vi "main.vi"() -> ()   [LabVIEW 2019]
uses:
  <vilib>/DAQmx/write.llb/DAQmx Write (Digital Wfm 1Chan NSamp).vi
  <vilib>/DAQmx/write.llb/DAQmx Write (Analog DBL 1Chan 1Samp).vi
  <vilib>/DAQmx/write.llb/DAQmx Write (Digital Bool 1Line 1Point).vi
  <userlib>/AndorSDK3/Data/GetPixelData16.vi
  <vilib>/DAQmx/create/channels.llb/DAQmx Create Channel (AO-Voltage-Basic).vi
  <vilib>/DAQmx/miscellaneous.llb/DAQmx Fill In Error Info.vi
  <vilib>/DAQmx/create/channels.llb/DAQmx Create Channel (DO-Digital Output).vi
  <vilib>/Utility/file.llb/Write Delimited Spreadsheet (DBL).vi
  <vilib>/DAQmx/configure/timing.llb/DAQmx Timing (Sample Clock).vi
  <vilib>/DAQmx/configure/trigger.llb/DAQmx Start Trigger (Digital Edge).vi
  <vilib>/Waveform/DWDTOps.llb/DWDT Uncompress Digital.vi
  <resource>/objmgr/daqmx.rc
panel:
  in  "show temperature":bool
  in  "Start.Retriggerable 2":bool
  in  "waveform generation 3":bool
  out "DO signal 2":dbl[][](array[numeric])
  in  "waveform generation 2":bool
  in  "waveform is generating":bool
  in  "Status":string
  out "acquired images 2":i32
  in  "free run save path":path
  in  "Tab Control 3":enum32{"sCMOS camera"}(tab)
  in  "ExposureTime (s)":dbl=0.1
  in  "PreAmp Gain Control":string(combo)
  in  "Live":bool
  in  "AOI Height":i64
  in  "AOI Width":i64
  in  "Centre AOI":bool
  in  "Apply Settings":bool
  in  "open/close camera":bool
  in  "Trigger mode":string(combo)
  in  "min_value":dbl
  in  "max_value":dbl
  in  "auto constrast":bool
  in  "ElectronicShutteringMode":string(combo)
  in  "Pixel Readout Rate":string(combo)="280 MHz"
  in  "save to disk":bool
  in  "Save path":path
  in  "Frame number":i32
  out "camera temperature(℃)":dbl
  in  "Tab Control 2":enum32{"Control"}(tab)
  out "rps":dbl format="%0.4f"
  in  "Stop/Start":bool
  in  "rotary voltage":dbl min=0.0 max=1.0 step=0.01 format="%0.4f"
  in  "DO Trigger Type":enum32{"No Trigger", "Digital Start"}(ring)
  in  "z position (mm)":dbl min=0.0 max=20.0 step=0.01
  out "T(ms)":dbl format="%0.4f"
  out "camclockfreq":i64
  out "MetaData":i64
  out "TimeStamp":dbl
  in  "Overlap":bool
  out "FrameRate":dbl
  out "get&save image disk":bool
  out "acquired images":i32
  out "dmd_picture_time":dbl
  in  "save parameter":bool
  out "parameters":dbl[](array[numeric])
  in  "Start.Retriggerable":bool
  out "call matlab for acq":bool
  out "call matlab for cali":bool
  out "dmd projection":bool
  out "memory allocated":bool
  in  "waveform generation":bool
  in  "pattern path":path
  in  "load patterns":bool
  in  "get&save image":bool
  out "DO signal":dbl[][](array[numeric])
  in  "String":string
  out "ALP_INVALID_ID":u32=4294967295
  out "saving":bool
  in  "image num":u64
  out "acquiring":bool
  out "previewing":bool
  out "Waveform Graph":dynamicdata(graph)
  out "camera image":T1(plugin-control)
  out "DMD return2":i32[](array[numeric])
  out "DMD return1":i32[](array[numeric])
  out "DMD DevId":u32
  out "DMD SeqId":u32
  in  "initializing":bool
  out "ready":bool
  in  "Error":errorcluster
  out "AOIStride":i64
  out "Pixel Encoding":string
  out "PixelData":u16[](array[numeric])
  out "ByteData":u8[](array[numeric])
  out "ImageSizeBytes":i64
  out "Handle":i32
  in  "z stage COM":refnum<visa-resource-name>
  out "DO sample num":i32=1000
  in  "DO trigger edge":i32(ring)=10280 items=["rising"=10280, "falling"=10171]
  in  "DO trigger channel":tag
  in  "DO channels":tag
  out "DMD pattern":T1(plugin-control)
  in  "Tab Control":enum32{"Free Run", "Calibration", "Acquisition"}(tab)
  in  "free run save":bool caption="Start 2"
  in  "DMD":bool
  in  "File Path":path
  in  "pattern type":u16(ring) items=["from file", "all 0", "all 1"]
  in  "LED":bool
  in  "waveform only":bool
  in  "load cali pattern":bool
  in  "cali pattern path":path
  in  "illumination delay deg":dbl
  in  "start cali":bool
  in  "signal time (ms)":dbl
  in  "cam delay deg":dbl
  in  "dmd delay deg":dbl
  in  "dmd pattern num":u64
  in  "illumination last deg":dbl
  in  "acq signal time (ms)":dbl
  in  "acq waveform only":bool
  in  "acq pattern path":path
  in  "start acq":bool
  in  "rotary in":tag
  in  "starting edge":i32(ring)=10280 items=["Rising"=10280, "Falling"=10171]
  out "sample rate":dbl=1000.0 format="%0.2f"
  in  "counter":tag="Dev1/ctr0"
  in  "rotary out":tag
  in  "Stop":bool
  # "intermediate variables"
  # "indicate that images should be directly saved to disk"
  # "indicate that 'start cali' or 'start acq' has been clicked"
  # "indicate that waveform should be started"
  # "if we want to load patterns on dmd"
  # "how many images will be acquired and saved"
  # "where the cali images and acq images are saved"
  # "where the dmd patterns are loaded"
  # "DO signal that will be generated"
  # "Rotary stage"
  # "Speed monitor"
  # "Z stage"
  # "DMD and camera trigger"
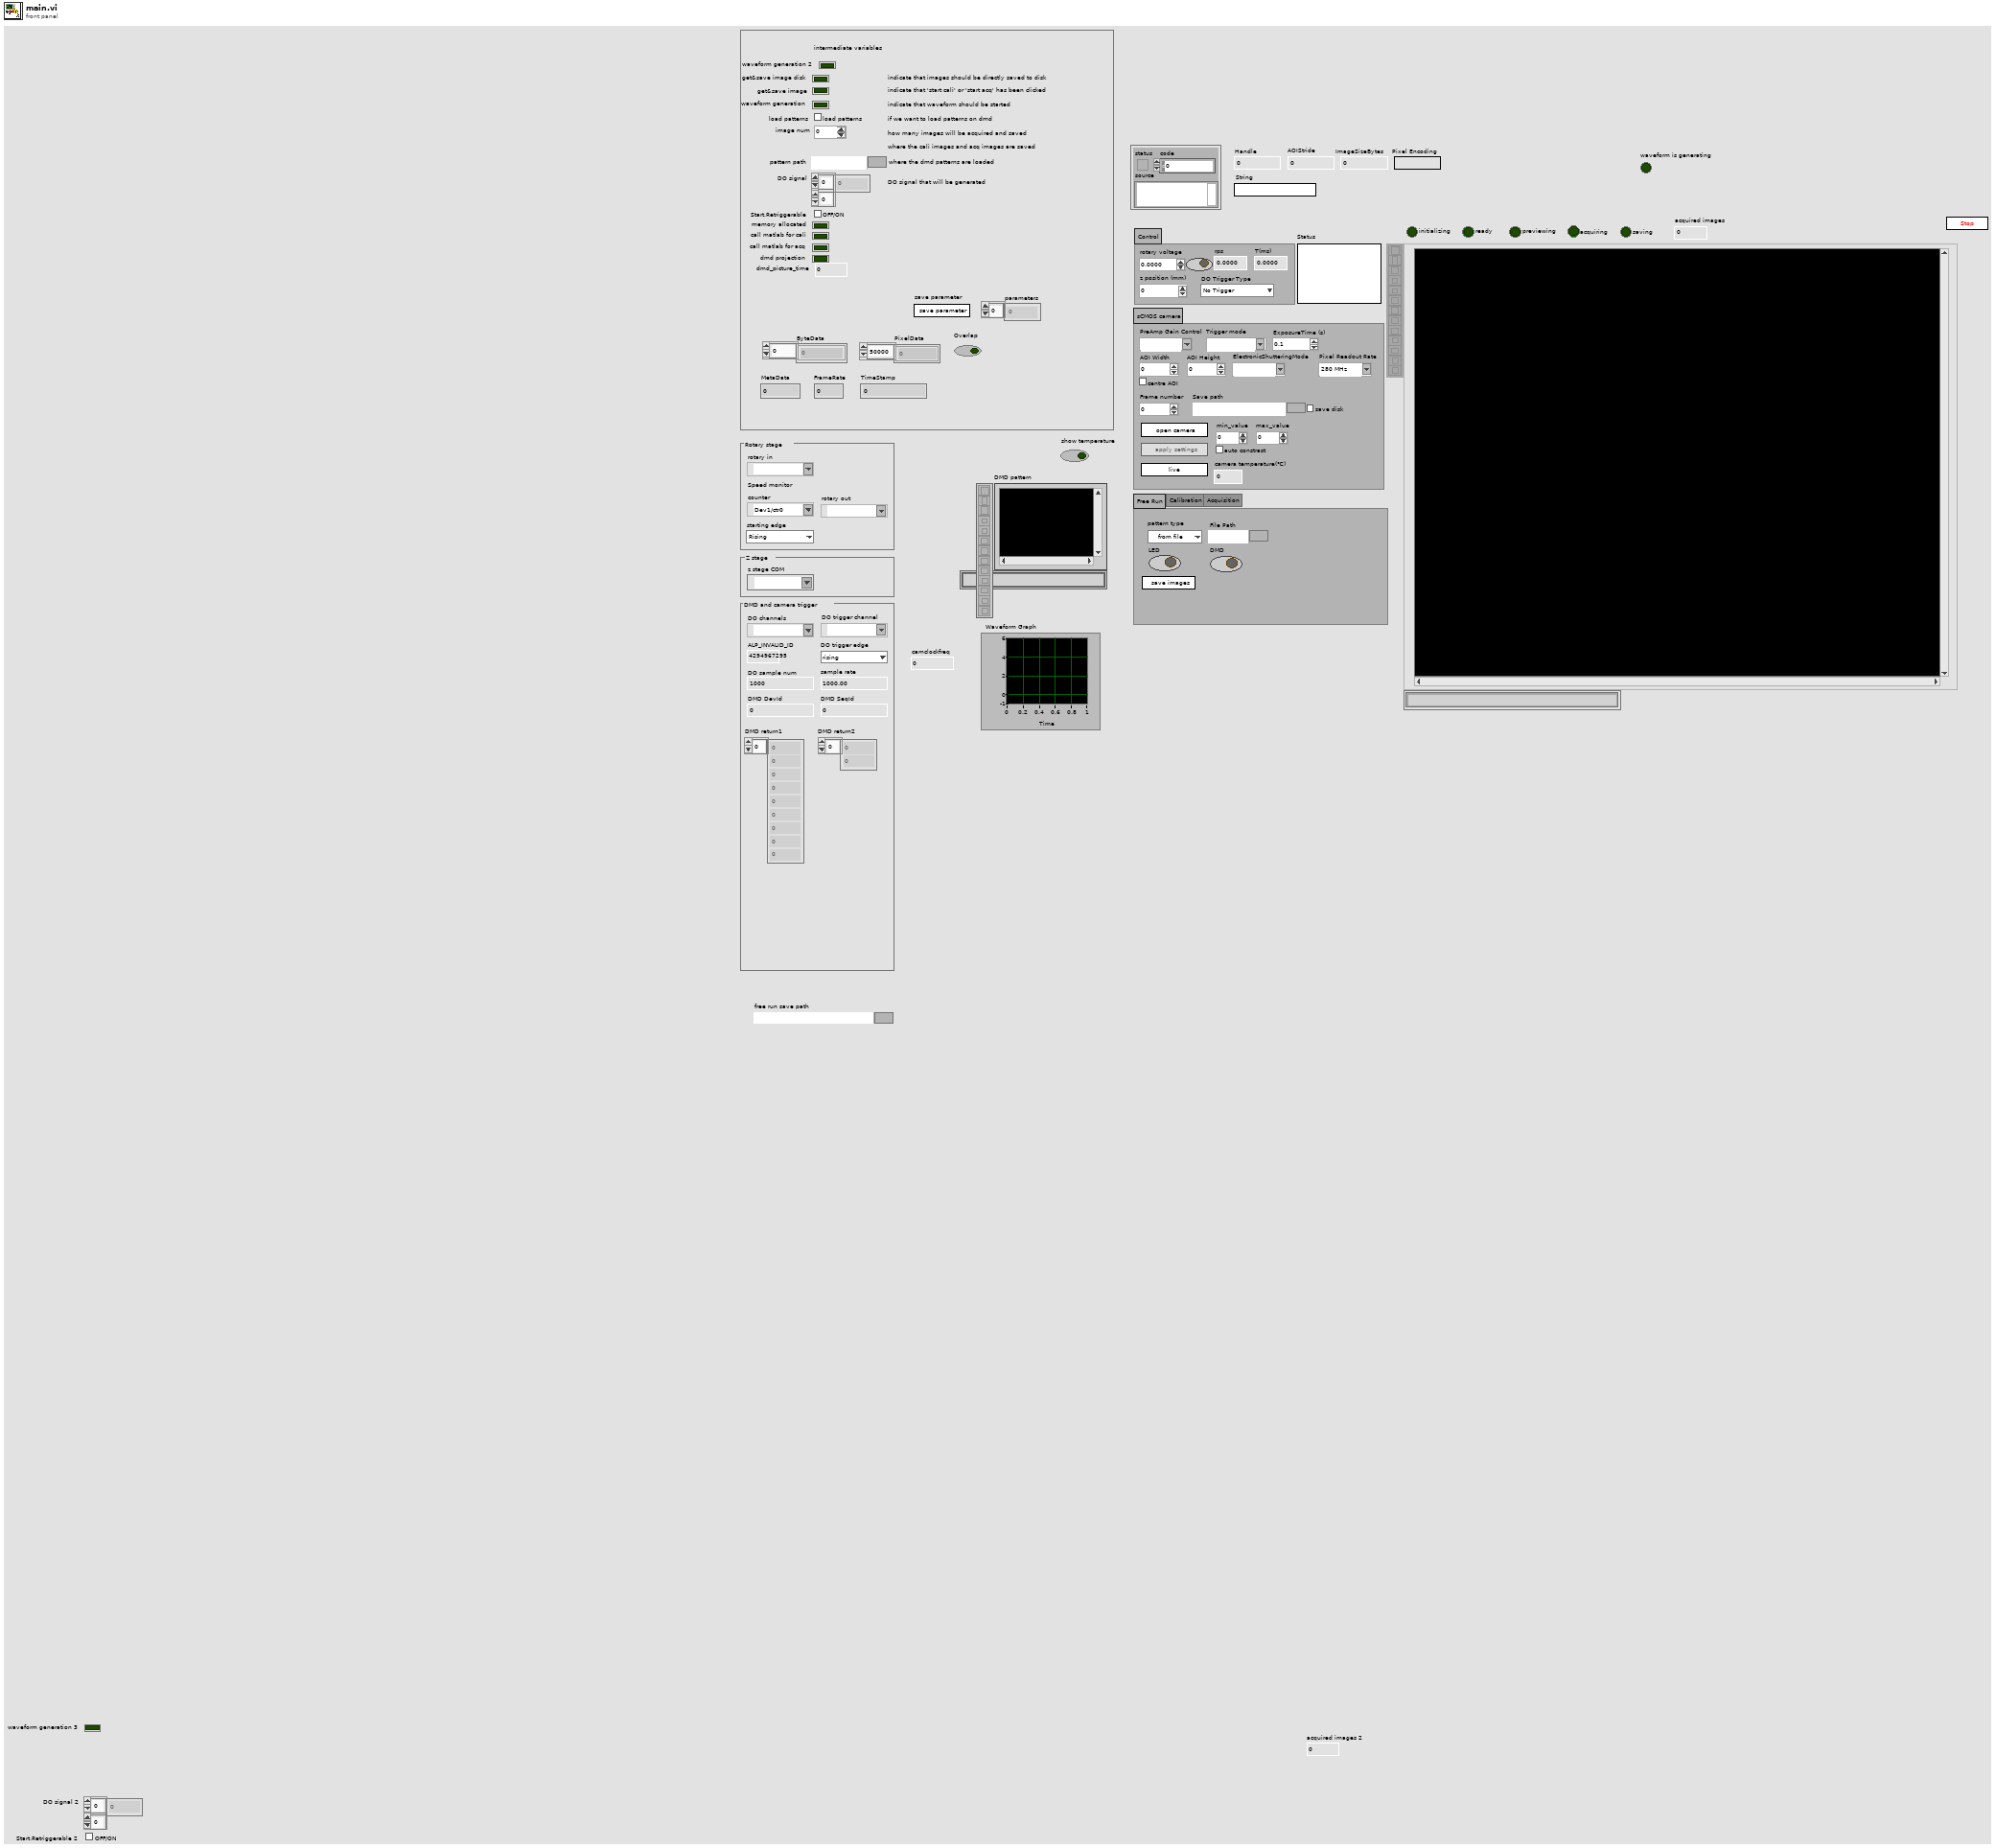
[diagram p1: front panel]
types:
  T1 = typedef "IMAQ Image.ctl" = refnum<image>
  T2 = enum8{"Enabled", "Disabled", "Disabled and Grayed Out"}
  T3 = typedef "Image Type" = u32
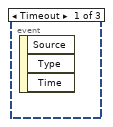
[diagram p3: hidden frame]
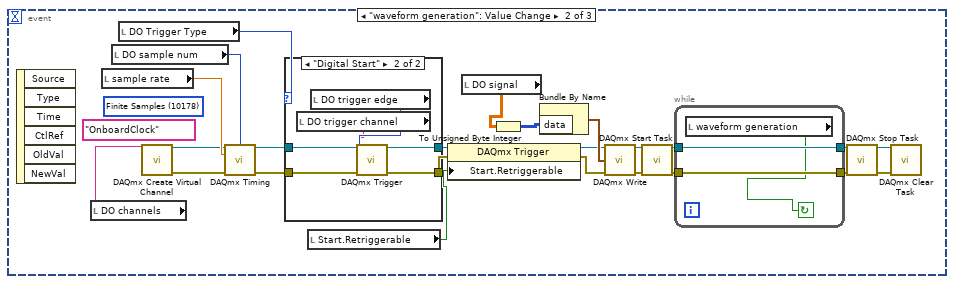
[diagram p4: hidden frame]
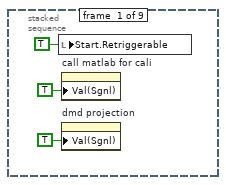
[diagram p7: hidden frame]
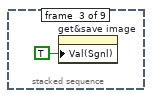
[diagram p8: hidden frame]
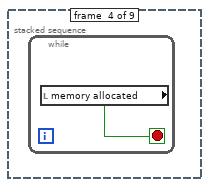
[diagram p9: hidden frame]
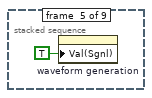
[diagram p10: hidden frame]
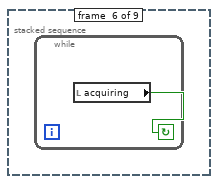
[diagram p11: hidden frame]
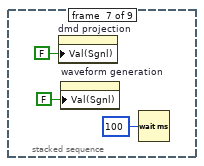
[diagram p12: hidden frame]
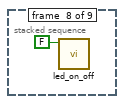
[diagram p13: hidden frame]
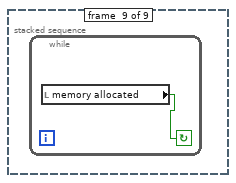
[diagram p14: hidden frame]
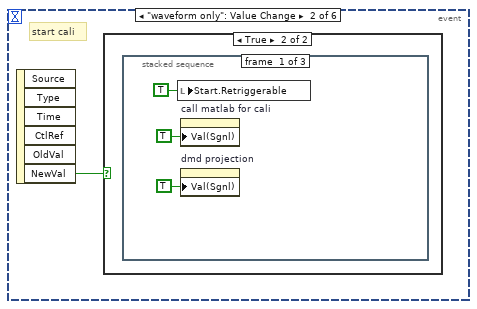
[diagram p15: hidden frame]
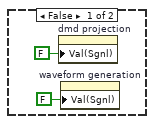
[diagram p16: hidden frame]
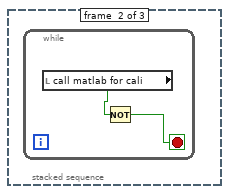
[diagram p17: hidden frame]
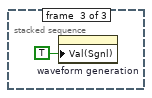
[diagram p18: hidden frame]
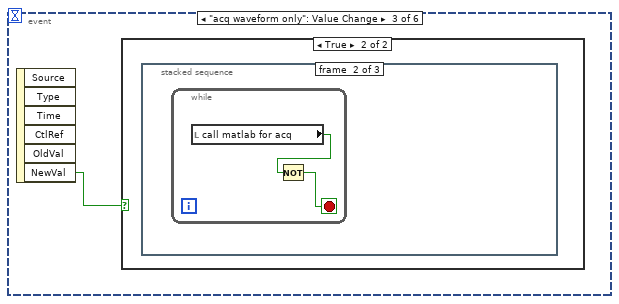
[diagram p19: hidden frame]
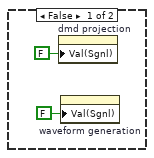
[diagram p20: hidden frame]
diagram:
  n1 = flat-sequence {
    frame #0 {
      w22 = T3 7 items=["Grayscale (U8)", "Grayscale (I16)", "Grayscale (SGL)", "Complex (CSG)", "RGB (U32)", "HSL (U32)", "RGB (U64)", "Grayscale (U16)"] ("Image Type")
      w11 = FALSE ("start button clicked")
      w28 = 10280 items=["rising"=10280, "falling"=10171] ("DO trigger edge")
      w33 = FALSE ("previewing")
      w35 = u16 2 items=["from file", "all 0", "all 1"] ("pattern type")
      w37 = tag "/Dev1/PFI9" ("转台输出通道")
      # "intermediate variables"
      # "acquisition"
      # "gui"
      # "Camera"
      # "Calibration"
      # "free run and dmd"
      # "triggers"
      # "z stage"
      # "rotary stage"
      n2 = Initialize Array(u16 0 ("element"), 2160 ("dimension size"), 2560 ("dimension size")) -> (w17:u16[][])
      n3 = call "IMAQ Create"("Image Name"="cam", "Image Type"=w22) -> ("New Image"=w21:T1)  [unwired: 3 in, 1 out]
      n4 = local read "ALP_INVALID_ID"() -> (w29:u32)
      n5 = call "IMAQ ArrayToImage"("Image Pixels (U16)"=w17, "Image"=w21) -> ("Image Out"=w16:T1)  [unwired: 8 in, 1 out]
      n6 = call <vilib>:"Application Directory.vi"() -> ("Application Directory"=w2:path)
      n7 = call <vilib>:"Application Directory.vi"() -> ("Application Directory"=w3:path)
      n8 = local write "illumination delay deg"(6.0 ("illumination delay deg")) -> ()
      n9 = local write "illumination last deg"(23.0 ("illumination last deg")) -> ()
      n10 = local write "Stop"(FALSE ("停止")) -> ()
      n11 = local write "sample rate"(1000.0 ("采样率")) -> ()
      n12 = local write "Stop/Start"(FALSE ("Stop/Start")) -> ()
      n13 = local write "dmd pattern num"(10.0 ("dmd pattern num")) -> ()
      n14 = local write "pattern type"(w35) -> ()
      n15 = local write "signal time (ms)"(500.0 ("fps")) -> ()
      n16 = Build Path(base path=w3, name or relative path=path "default_image_path/default_save_path" ("cali save path")) -> (appended path=w6:path)
      n17 = Build Path(base path=w2, name or relative path=path "default_image_path/acq_patterns" ("cali pattern path")) -> (appended path=w8:path)
      n18 = local write "z stage COM"(refnum<visa-resource-name> "COM3" ("z stage COM")) -> ()
      n19 = local write "DO trigger edge"(w28) -> ()
      n20 = local write "camera image"(w16) -> ()
      n21 = property on="DMD" class="Bool (strict)"("DisabledEnum"=T2."Enabled" ("Disabled")) -> ()  [unwired: 2 in, 2 out]
      n22 = local write "DO trigger channel"(w37) -> ()
      n23 = local write "cali pattern path"(w8) -> ()
      n24 = local write "rotary out"(w37) -> ()
      n25 = local write "DMD DevId"(w29) -> ()
      n26 = local write "DO Trigger Type"(enum32{"No Trigger", "Digital Start"}."Digital Start" ("DO Trigger Type")) -> ()
      n27 = local write "Save path"(w6) -> ()
      n28 = local write "DO channels"(tag "Dev1/port0/line0:2" ("DO channels")) -> ()
      n29 = local write "rotary in"(tag "Dev1/ao1" ("rotary voltage channel")) -> ()
      n30 = call <vilib>:"Application Directory.vi"() -> ("Application Directory"=w1:path)
      n31 = Build Path(base path=w1, name or relative path=path "default_image_path/acq_patterns" ("cali pattern path")) -> (appended path=w4:path)
      n32 = local write "ExposureTime (s)"(0.01 ("ExposureTime (s)")) -> ()
      n33 = local write "previewing"(w33) -> ()
      n34 = local write "acquiring"(w33) -> ()
      n35 = local write "max_value"(1000.0 ("max_value")) -> ()
      n36 = local write "waveform generation"(w11) -> ()
      n37 = local write "min_value"(0.0 ("min_value")) -> ()
      n38 = local write "Frame number"(10 ("free run frame number")) -> ()
      n39 = local write "get&save image disk"(w11) -> ()
      n40 = local write "show temperature"(FALSE ("show temperature")) -> ()
      n41 = local write "get&save image"(w11) -> ()
      n42 = local write "Tab Control"(enum32{"Free Run", "Calibration", "Acquisition"}."Free Run" ("Tab Control")) -> ()
      n43 = local write "acq pattern path"(w4) -> ()
      n44 = local write "ElectronicShutteringMode"("Global" ("ElectronicShutteringMode")) -> ()
      n45 = local write "Trigger mode"("Software" ("Trigger mode")) -> ()
      "ALP_INVALID_ID" <- u32 4294967295
    }
    frame #1 {
      n46 = while {
        stop <- w52 stop-if-true
        # "waveform for different acquisition"
        n47 = event shown="[2] \"waveform generation 2\": Value Change" {
          selector: _ -> [_ _ _]
          dyn-events: _ -> [_ _ _]
          timeout: 1 -> [_ _ _]
          event Timeout {
            n48 = event-data() -> ()  [unwired: 1 in, 3 out]
          }
          event "waveform generation": Value Change {
            (unwired) 10178 items=["Finite Samples"=10178, "Continuous Samples"=10123, "Hardware Timed Single Point"=12522] ("sample mode")
            (unwired) tag "OnboardClock" ("采样时钟源")
            n49 = event-data() -> ()  [unwired: 1 in, 6 out]
            n50 = local read "DO channels"() -> (w72:tag)
            n51 = local read "sample rate"() -> (w76:dbl)
            n52 = local read "DO sample num"() -> (w75:i32)
            n53 = local read "DO Trigger Type"() -> (w63:enum32{"No Trigger", "Digital Start"})
            n54 = call-poly <vilib>:"DAQmx Create Virtual Channel.vi"("lines"=w72) -> ("task out"=w64:refnum<k21>, "error out"=w65:errorcluster)  [unwired: 13 in]
            n55 = call-poly <vilib>:"DAQmx Timing.vi"("task/channels in"=w64, "samples per channel"=w75, "rate"=w76, "error in"=w65) -> ("task out"=w66:refnum<k21>, "error out"=w67:errorcluster)  [unwired: 10 in]
            n56 = case shown="\"Digital Start\"" w63 {
              tunnel: w66 -> [w81 w87]
              tunnel: w67 -> [w80 w86]
              tunnel: [w81 w85] -> w62
              tunnel: [w80 w84] -> w61
              frame "No Trigger", Default {
              }
              frame "Digital Start" {
                n57 = local read "DO trigger channel"() -> (w82:tag)
                n58 = local read "DO trigger edge"() -> (w83:i32)
                n59 = call-poly <vilib>:"DAQmx Trigger.vi"("task/channels in"=w87, "source"=w82, "edge"=w83, "error in"=w86) -> ("task out"=w85:refnum<k21>, "error out"=w84:errorcluster)  [unwired: 10 in]
              }
            }
            n60 = local read "Start.Retriggerable"() -> (w53:bool)
            n61 = property class="DAQmx Trigger"(reference=w62, error in=w61, "Start.Retriggerable"=w53) -> (reference out=w60:refnum<k21>, error out=w59:errorcluster)
            n62 = local read "DO signal"() -> (w54:dbl[][])
            n63 = To Unsigned Byte Integer(number=w54) -> (unsigned 8bit integer=w73:u8[][])
            n64 = Bundle By Name("data"=w73) -> (w74:digitaldata)  [unwired: 1 in]
            n65 = call-poly <vilib>:"DAQmx Write.vi"("task/channels in"=w60, "data"=w74, "error in"=w59) -> ("task out"=w68:refnum<k21>, "error out"=w69:errorcluster)  [unwired: 10 in, 1 out]
            n66 = call <vilib>:"DAQmx Start Task.vi"("task/channels in"=w68, "error in"=w69) -> ("task out"=w58:refnum<k21>, "error out"=w56:errorcluster)  [unwired: 12 in]
            n67 = while {
              tunnel: w58 -> [w79]
              tunnel: [w79] -> w57
              tunnel: w56 -> [w78]
              tunnel: [w78] -> w55
              stop <- w77 continue-if-true
              n68 = local read "waveform generation"() -> (w77:bool)
            }
            n69 = call <vilib>:"DAQmx Stop Task.vi"("task/channels in"=w57, "error in"=w55) -> ("task out"=w70:refnum<k21>, "error out"=w71:errorcluster)  [unwired: 12 in]
            n70 = call <vilib>:"DAQmx Clear Task.vi"("task in"=w70, "error in"=w71) -> ()  [unwired: 13 in, 1 out]
          }
          event "waveform generation 2": Value Change {
            w98 = 10178 items=["Finite Samples"=10178, "Continuous Samples"=10123, "Hardware Timed Single Point"=12522] ("sample mode")
            n71 = event-data() -> ()  [unwired: 1 in, 6 out]
            n72 = local read "DO channels"() -> (w105:tag)
            n73 = local read "sample rate"() -> (w109:dbl)
            n74 = local read "DO sample num"() -> (w108:i32)
            n75 = call-poly <vilib>:"DAQmx Create Virtual Channel.vi"("lines"=w105) -> ("task out"=w99:refnum<k21>, "error out"=w100:errorcluster)  [unwired: 13 in]
            n76 = call-poly <vilib>:"DAQmx Timing.vi"("task/channels in"=w99, "sample mode"=w98, "samples per channel"=w108, "rate"=w109, "source"=tag "OnboardClock" ("采样时钟源"), "error in"=w100) -> ("task out"=w94:refnum<k21>, "error out"=w93:errorcluster)  [unwired: 8 in]
            n77 = local read "DO signal"() -> (w96:dbl[][])
            n78 = To Unsigned Byte Integer(number=w96) -> (unsigned 8bit integer=w106:u8[][])
            n79 = Bundle By Name("data"=w106) -> (w107:digitaldata)  [unwired: 1 in]
            n80 = call-poly <vilib>:"DAQmx Write.vi"("task/channels in"=w94, "data"=w107, "error in"=w93) -> ("task out"=w101:refnum<k21>, "error out"=w102:errorcluster)  [unwired: 10 in, 1 out]
            n81 = call <vilib>:"DAQmx Start Task.vi"("task/channels in"=w101, "error in"=w102) -> ("task out"=w92:refnum<k21>, "error out"=w91:errorcluster)  [unwired: 12 in]
            n82 = local write "waveform is generating"(TRUE ("Boolean")) -> ()
            n83 = call <vilib>:"DAQmx Wait Until Done.vi"("task/channels in"=w92, "timeout (sec)"=200.0, "error in"=w91) -> ("task out"=w90:refnum<k21>, "error out"=w89:errorcluster)  [unwired: 11 in]
            n84 = call <vilib>:"DAQmx Stop Task.vi"("task/channels in"=w90, "error in"=w89) -> ("task out"=w103:refnum<k21>, "error out"=w104:errorcluster)  [unwired: 12 in]
            n85 = call <vilib>:"DAQmx Clear Task.vi"("task in"=w103, "error in"=w104) -> ()  [unwired: 13 in, 1 out]
          }
        }
        n86 = local read "Stop"() -> (w52:bool)
      }
      n87 = while {
        stop <- w208 stop-if-true
        # "control rotary stage, z stage, free run led, free run dmd, tab change"
        n88 = event shown="[3] \"LED\": Value Change" {
          selector: _ -> [_ _ _ _ _ _ _ _ _]
          dyn-events: _ -> [_ _ _ _ _ _ _ _ _]
          timeout: 1 -> [_ _ _ _ _ _ _ _ _]
          event Timeout {
            n89 = event-data() -> ()  [unwired: 1 in, 3 out]
          }
          event "dmd projection": Value Change {
            n90 = event-data() -> ("NewVal"=w210:bool)  [unwired: 1 in, 5 out]
            n91 = case shown="False" w210 {
              frame False {
                n92 = local read "DMD DevId"() -> (w211:u32)
                n93 = local read "ALP_INVALID_ID"() -> (w213:u32)
                n94 = call "stop_and_free_dmd.vi"("DevId"=w211) -> ("return array2"=w212:i32[])  [unwired: 10 in]
                n95 = local write "DMD return2"(w212) -> ()
                n96 = local write "DMD DevId"(w213) -> ()
              }
              frame True {
                # "project patterns"
                n97 = local read "dmd_picture_time"() -> (w214:dbl)
                n98 = local read "load patterns"() -> (w217:bool)
                n99 = local read "pattern path"() -> (w215:path)
                n100 = call "alloc_and_project_patterns_dmd.vi"("Path"=w215, "PicNum"=10, "load patterns"=w217, "PictureTime"=w214) -> ("return array"=w218:i32[], "SeqId"=w219:u32, "DevId"=w220:u32)  [unwired: 5 in]
                n101 = local write "DMD return1"(w218) -> ()
                n102 = local write "DMD DevId"(w220) -> ()
                n103 = local write "DMD SeqId"(w219) -> ()
              }
            }
          }
          event "rotary voltage": Value Change {
            # "use a AO task to change the stage speed"
            n104 = event-data() -> ()  [unwired: 1 in, 6 out]
            n105 = local read "rotary in"() -> (w222:tag)
            n106 = call <vilib>:"DAQmx Create Task.vi"() -> ("task out"=w233:refnum<k21>, "error out"=w232:errorcluster)  [unwired: 14 in]
            n107 = call-poly <vilib>:"DAQmx Create Virtual Channel.vi"("task in"=w233, "maximum value"=1.0, "minimum value"=0.0, "physical channels"=w222, "error in"=w232) -> ("task out"=w231:refnum<k21>)  [unwired: 9 in, 1 out]
            n108 = local read "rotary voltage"() -> (w221:dbl)
            n109 = call-poly <vilib>:"DAQmx Write.vi"("task/channels in"=w231, "data"=w221) -> ("task out"=w230:refnum<k21>, "error out"=w229:errorcluster)  [unwired: 11 in, 1 out]
            n110 = call <vilib>:"DAQmx Start Task.vi"("task/channels in"=w230, "error in"=w229) -> ("task out"=w228:refnum<k21>, "error out"=w227:errorcluster)  [unwired: 12 in]
            n111 = call <vilib>:"DAQmx Stop Task.vi"("task/channels in"=w228, "error in"=w227) -> ("task out"=w226:refnum<k21>, "error out"=w225:errorcluster)  [unwired: 12 in]
            n112 = call <vilib>:"DAQmx Clear Task.vi"("task in"=w226, "error in"=w225) -> ()  [unwired: 13 in, 1 out]
          }
          event "LED": Value Change {
            w244 = TRUE  # auto start
            # "use DO output to control LED"
            n113 = event-data() -> ()  [unwired: 1 in, 6 out]
            n114 = call <vilib>:"DAQmx Create Task.vi"("auto cleanup"=TRUE) -> ("task out"=w248:refnum<k21>, "error out"=w247:errorcluster)  [unwired: 13 in]
            n115 = call-poly <vilib>:"DAQmx Create Virtual Channel.vi"("task in"=w248, "lines"=tag "Dev1/port0/line2", "error in"=w247) -> ("task out"=w240:refnum<k21>, "error out"=w239:errorcluster)  [unwired: 11 in]
            n116 = call <vilib>:"DAQmx Start Task.vi"("task/channels in"=w240, "error in"=w239) -> ("task out"=w246:refnum<k21>, "error out"=w245:errorcluster)  [unwired: 12 in]
            n117 = local read "LED"() -> (w235:bool)
            n118 = call-poly <vilib>:"DAQmx Write.vi"("task/channels in"=w246, "auto start"=w244, "data"=w235, "timeout"=10.0, "error in"=w245) -> ("task out"=w243:refnum<k21>, "error out"=w242:errorcluster)  [unwired: 8 in, 1 out]
            n119 = call <vilib>:"DAQmx Stop Task.vi"("task/channels in"=w243, "error in"=w242) -> ("task out"=w237:refnum<k21>, "error out"=w238:errorcluster)  [unwired: 12 in]
            n120 = call <vilib>:"DAQmx Clear Task.vi"("task in"=w237, "error in"=w238) -> ()  [unwired: 13 in, 1 out]
          }
          event "DMD": Value Change {
            n121 = event-data() -> ("NewVal"=w249:bool)  [unwired: 1 in, 5 out]
            n122 = case shown="True" w249 {
              frame False {
                n123 = flat-sequence {
                  frame #0 {
                    n124 = local read "DMD DevId"() -> (w251:u32)
                    n125 = call "stop_and_free_dmd.vi"("DevId"=w251) -> ("return array2"=w250:i32[])  [unwired: 10 in]
                    n126 = local write "DMD return2"(w250) -> ()
                  }
                  frame #1 {
                    n127 = local read "ALP_INVALID_ID"() -> (w252:u32)
                    n128 = local write "DMD DevId"(w252) -> ()
                  }
                }
              }
              frame True {
                n129 = local read "pattern type"() -> (w257:u16)
                n130 = local read "File Path"() -> (w258:path)
                n131 = call "alloc_and_project_single_pattern_dmd.vi"("pattern type"=w257, "File Path"=w258) -> ("return array"=w253:i32[], "SeqId"=w254:u32, "DevId"=w255:u32, "Image Out"=w256:T1)  [unwired: 6 in]
                n132 = local write "DMD pattern"(w256) -> ()
                n133 = local write "DMD DevId"(w255) -> ()
                n134 = local write "DMD SeqId"(w254) -> ()
                n135 = local write "DMD return1"(w253) -> ()
              }
            }
          }
          event "save parameter": Value Change {
            n136 = event-data() -> ()  [unwired: 1 in, 6 out]
            n137 = local read "dmd pattern num"() -> (w264:u64)
            n138 = local read "signal time (ms)"() -> (w263:dbl)
            n139 = local read "z position (mm)"() -> (w262:dbl)
            n140 = local read "rotary voltage"() -> (w261:dbl)
            n141 = Build Array(w262, w261, w263, w264) -> (w265:dbl[])
            n142 = call-poly <vilib>:"Write Delimited Spreadsheet.vi"("file path (dialog if empty)"=path "D:/widefield_surface_imaging/parameters.csv", "1D data"=w265, "append to file? (new file:F)"=FALSE) -> ()  [unwired: 11 in, 2 out]
          }
          event "Tab Control": Value Change {
            n143 = event-data() -> ("NewVal"=w269:enum32{"Free Run", "Calibration", "Acquisition"})  [unwired: 1 in, 5 out]
            n144 = local read "ALP_INVALID_ID"() -> (w267:u32)
            n145 = local read "DMD DevId"() -> (w268:u32)
            n146 = case shown="\"Calibration\"" w269 {
              frame "Free Run", Default {
                n147 = local write "Trigger mode"("Software" ("Trigger mode")) -> ()
              }
              frame "Calibration" {
                n148 = local write "save to disk"(FALSE ("save to disk")) -> ()
                n149 = property on="call matlab for cali" class="Bool (strict)"("Val(Sgnl)"=TRUE ("Value (Signaling)")) -> ()  [unwired: 2 in, 2 out]
                n150 = local write "Trigger mode"("External" ("Trigger mode")) -> ()
              }
              frame "Acquisition" {
                n151 = property on="call matlab for acq" class="Bool (strict)"("Val(Sgnl)"=TRUE ("Value (Signaling)")) -> ()  [unwired: 2 in, 2 out]
                n152 = local write "Trigger mode"("External" ("Trigger mode")) -> ()
              }
            }
            n153 = Not Equal?(x=w268, y=w267) -> (x != y?=w266:bool)
            n154 = case shown="True" w266 {
              frame False {
              }
              frame True {
                n155 = local read "DMD DevId"() -> (w272:u32)
                n156 = local read "ALP_INVALID_ID"() -> (w270:u32)
                n157 = call "stop_and_free_dmd.vi"("DevId"=w272) -> ("return array2"=w271:i32[])  [unwired: 10 in]
                n158 = local write "DMD DevId"(w270) -> ()
                n159 = local write "DMD return2"(w271) -> ()
              }
            }
          }
          event "signal time (ms)", "dmd pattern num", "cam delay deg", "dmd delay deg", "illumination last deg", "illumination delay deg": Value Change {
            n160 = event-data() -> ()  [unwired: 1 in, 6 out]
            n161 = property on="call matlab for cali" class="Bool (strict)"("Val(Sgnl)"=TRUE ("Value (Signaling)")) -> ()  [unwired: 2 in, 2 out]
          }
          event "acq signal time (ms)": Value Change {
            n162 = event-data() -> ()  [unwired: 1 in, 6 out]
            n163 = property on="call matlab for acq" class="Bool (strict)"("Val(Sgnl)"=TRUE ("Value (Signaling)")) -> ()  [unwired: 2 in, 2 out]
          }
        }
        n164 = local read "Stop"() -> (w208:bool)
      }
      n165 = while {
        stop <- w281 stop-if-true
        # "preview and get images"
        n166 = event shown="[4] \"get&save image\": Value Change" {
          selector: _ -> [_ _ _ _ _ _]
          dyn-events: _ -> [_ _ _ _ _ _]
          timeout: 1 -> [_ _ _ _ _ _]
          event Timeout {
            n167 = event-data() -> ()  [unwired: 1 in, 3 out]
          }
          event "open/close camera": Value Change {
            n168 = event-data() -> ("NewVal"=w283:bool)  [unwired: 1 in, 5 out]
            n169 = case shown="False" w283 {
              frame False {
                n170 = flat-sequence {
                  frame #0 {
                    n171 = local write "show temperature"(FALSE ("show temperature")) -> ()
                  }
                  frame #1 {
                    # "ShutDown."
                    n172 = local read "Handle"() -> (w285:i32)
                    n173 = call "close_camera.vi"("Handle"=w285) -> ()  [unwired: 11 in]
                  }
                  frame #2 {
                    n174 = local write "ready"(FALSE ("Ready")) -> ()
                    n175 = property on="Apply Settings" class="Bool (strict)"("DisabledEnum"=T2."Disabled and Grayed Out" ("Disabled")) -> ()  [unwired: 2 in, 2 out]
                  }
                }
              }
              frame True {
                n176 = flat-sequence {
                  frame #0 {
                    n177 = call "open_camera.vi"() -> ("error"=w294:errorcluster, "AOI Height"=w293:i64, "AOI Width"=w292:i64, "Handle"=w291:i32, "PreAmp Gain Control"=w295:string)  [unwired: 7 in]
                    n178 = local write "initializing"(TRUE ("Initializing")) -> ()
                    n179 = local write "PreAmp Gain Control"(w295) -> ()
                    n180 = local write "Live"(FALSE ("Run")) -> ()
                    n181 = local write "Handle"(w291) -> ()
                    n182 = local write "AOI Width"(w292) -> ()
                    n183 = local write "AOI Height"(w293) -> ()
                    n184 = local write "Error"(w294) -> ()
                    n185 = property on="Live" class="Bool (strict)"("DisabledEnum"=T2."Disabled and Grayed Out" ("Disabled")) -> ()  [unwired: 2 in, 2 out]
                  }
                  frame #1 {
                    n186 = local write "show temperature"(TRUE ("show temperature")) -> ()
                    n187 = local write "initializing"(FALSE ("Initializing")) -> ()
                    n188 = local write "ready"(TRUE ("Ready")) -> ()
                    n189 = property on="Apply Settings" class="Bool (strict)"("DisabledEnum"=T2."Enabled" ("Disabled")) -> ()  [unwired: 2 in, 2 out]
                  }
                }
              }
            }
          }
          event "Apply Settings": Value Change {
            n190 = event-data() -> ()  [unwired: 1 in, 6 out]
            n191 = flat-sequence {
              frame #0 {
                n192 = local read "ElectronicShutteringMode"() -> (w300:string)
                n193 = local read "PreAmp Gain Control"() -> (w307:string)
                n194 = local read "Trigger mode"() -> (w306:string)
                n195 = local read "ExposureTime (s)"() -> (w312:dbl)
                n196 = local read "Centre AOI"() -> (w308:bool)
                n197 = local read "AOI Height"() -> (w310:i64)
                n198 = local read "AOI Width"() -> (w309:i64)
                n199 = local read "Handle"() -> (w311:i32)
                n200 = call "apply_settings.vi"("Handle"=w311, "PreAmp Gain Control"=w307, "Trigger mode"=w306, "ExposureTime"=w312, "ElectronicShutteringMode"=w300, "AOI Height"=w310, "AOI Width"=w309, "Centre AOI"=w308) -> ("AOIStride"=w305:i64, "ImageSizeBytes"=w304:i64, "Pixel Encoding"=w303:string, "PixelData"=w301:u16[], "ByteData"=w302:u8[])  [unwired: 3 in]
                n201 = local write "AOIStride"(w305) -> ()
                n202 = local write "ImageSizeBytes"(w304) -> ()
                n203 = local write "Pixel Encoding"(w303) -> ()
                n204 = local write "ByteData"(w302) -> ()
                n205 = local write "PixelData"(w301) -> ()
              }
              frame #1 {
                n206 = local write "Apply Settings"(FALSE ("Apply Settings")) -> ()
                n207 = property on="Live" class="Bool (strict)"("DisabledEnum"=T2."Enabled" ("Disabled")) -> ()  [unwired: 2 in, 2 out]
                n208 = local write "ready"(TRUE ("Ready")) -> ()
              }
            }
          }
          event "Live": Value Change {
            n209 = event-data() -> ("NewVal"=w316:bool)  [unwired: 1 in, 5 out]
            n210 = case shown="True" w316 {
              frame False {
                n211 = flat-sequence {
                  frame #0 {
                    # "Stop an acquisition if still running"
                    n212 = local read "Handle"() -> (w318:i32)
                    n213 = call <userlib>:"AT Command A.vi"("Feature"="AcquisitionStop" ("Command"), "Handle"=w318) -> ()  [unwired: 8 in, 2 out]
                  }
                  frame #1 {
                    # "re-enable controls"
                    n214 = local write "previewing"(FALSE ("previewing")) -> ()
                    n215 = property on="Apply Settings" class="Bool (strict)"("DisabledEnum"=T2."Enabled" ("Disabled")) -> ()  [unwired: 2 in, 2 out]
                  }
                }
              }
              frame True {
                w322 = "AcquisitionStart"  # Command
                # "Start the acquisition"
                # "Acquire"
                n216 = local read "Handle"() -> (w324:i32)
                n217 = local read "Error"() -> (w323:errorcluster)
                n218 = call <userlib>:"AT Command A.vi"("error in (no error)"=w323, "Feature"=w322, "Handle"=w324) -> ("error out"=w321:errorcluster)  [unwired: 7 in, 1 out]
                n219 = local write "Error"(w321) -> ()
                n220 = while {
                  tunnel: w324 -> [w328]
                  tunnel: w321 -> [w329]
                  stop <- w327 continue-if-true
                  # "This loop will continiously acquire data from the camera"
                  n221 = flat-sequence {
                    tunnel: w329 -> [w338]
                    tunnel: w328 -> [w339]
                    tunnel: [w330] -> w326
                    tunnel: w326 -> [w344]
                    tunnel: [w343] -> w325
                    tunnel: w325 -> [w353]
                    frame #0 {
                      # "Requeue the buffer\nfor the next image"
                      # "Send a trigger to the camera"
                      # "wait for the acquisition to \nreturn and retrieve the output"
                      n222 = call <userlib>:"AT Command A.vi"("error in (no error)"=w338, "Feature"="SoftwareTrigger" ("Command"), "Handle"=w339) -> ("error out"=w337:errorcluster)  [unwired: 7 in, 1 out]
                      n223 = local write "Error"(w337) -> ()
                      n224 = local read "ImageSizeBytes"() -> (w335:i64)
                      n225 = call <userlib>:"AT Wait Buffer A.vi"("error in (no error)"=w337, "Input buffer"=u32 0, "Timeout"=u32 10000, "Handle"=w339) -> ("error out"=w333:errorcluster, "Output buffer"=w332:u64)  [unwired: 4 in, 2 out]
                      n226 = local write "Error"(w333) -> ()
                      n227 = local read "ByteData"() -> (w336:u8[])
                      n228 = call <userlib>:"PointerToArrayEX.vi"("Array in"=w336, "Pointer In"=w332, "Pointer Size"=w335, "error in (no error)"=w333) -> ("Array out"=w331:u8[], "error out"=w334:errorcluster)  [unwired: 4 in]
                      n229 = local write "ByteData"(w331) -> ()
                      n230 = call <userlib>:"AT Queue Buffer A.vi"("error in (no error)"=w334, "PtrSize"=w335, "Ptr"=w332, "Handle"=w339) -> ("error out"=w330:errorcluster)  [unwired: 6 in, 1 out]
                      n231 = local write "Error"(w330) -> ()
                    }
                    frame #1 {
                      # "Convert the buffer containing byte \ndata into an array of pixels"
                      n232 = local read "Pixel Encoding"() -> (w350:string)
                      n233 = local read "AOI Height"() -> (w347:i64)
                      n234 = local read "AOI Width"() -> (w348:i64)
                      n235 = local read "AOIStride"() -> (w351:i64)
                      n236 = local read "ByteData"() -> (w345:u8[])
                      n237 = local read "PixelData"() -> (w349:u16[])
                      n238 = call-poly <userlib>:"GetPixelData.vi"("Input buffer"=w345, "Output buffer in"=w349, "Pixel Encoding"=w350, "Stride"=w351, "error in (no error)"=w344, "Width"=w348, "Height"=w347) -> ("Output buffer out"=w343:u16[], "error out"=w346:errorcluster)  [unwired: 10 in, 1 out]
                      n239 = local write "Error"(w346) -> ()
                    }
                    frame #2 {
                      w356 = T3 7 items=["Grayscale (U8)", "Grayscale (I16)", "Grayscale (SGL)", "Complex (CSG)", "RGB (U32)", "HSL (U32)", "RGB (U64)", "Grayscale (U16)"] ("Image Type")
                      # "Draw the image"
                      n240 = local read "AOI Height"() -> (w361:i64)
                      n241 = local read "AOI Width"() -> (w360:i64)
                      n242 = local read "auto constrast"() -> (w354:bool)
                      n243 = Reshape Array(w353, w361, w360) -> (w352:u16[][])
                      n244 = case shown="False" w354 {
                        tunnel: [w365 w366] -> w355
                        tunnel: w352 -> [w362 w366]
                        frame False {
                          n245 = local read "min_value"() -> (w364:dbl)
                          n246 = local read "max_value"() -> (w363:dbl)
                          n247 = call "set_min_max.vi"("max_value"=w363, "min_value"=w364, "array_in"=w362) -> ("array_out"=w365:u16[][])  [unwired: 8 in]
                        }
                        frame True {
                        }
                      }
                      n248 = call "IMAQ Create"("Image Name"="cam", "Image Type"=w356) -> ("New Image"=w357:T1)  [unwired: 3 in, 1 out]
                      n249 = call "IMAQ ArrayToImage"("Image Pixels (U16)"=w355, "Image"=w357) -> ("Image Out"=w359:T1)  [unwired: 8 in, 1 out]
                      n250 = local write "camera image"(w359) -> ()
                    }
                  }
                  n251 = local read "Live"() -> (w327:bool)
                  n252 = local write "previewing"(w327) -> ()
                }
              }
            }
          }
          event "get&save image": Value Change {
            n253 = event-data() -> ()  [unwired: 1 in, 6 out]
            n254 = stacked-sequence {
              seq-local: [w370 _ _ _] -> [_ _ w382 _]
              seq-local: [w367 _ _ _] -> [_ _ _ _]
              frame #0 {
                # "allocate memory"
                n255 = local read "image num"() -> (w369:u64)
                n256 = local read "AOI Height"() -> (w373:i64)
                n257 = local read "AOI Width"() -> (w372:i64)
                n258 = Initialize Array(u16 0 ("element"), w369, w373, w372) -> (w370:u16[][][])
                n259 = Initialize Array(0.0 ("element"), w369) -> (w367:dbl[])
              }
              frame #1 {
                n260 = flat-sequence {
                  frame #0 {
                    w379 = "AcquisitionStart"  # Command
                    # "Start the acquisition"
                    n261 = local read "Handle"() -> (w375:i32)
                    n262 = call <userlib>:"AT Command A.vi"("Feature"=w379, "Handle"=w375) -> ("error out"=w378:errorcluster)  [unwired: 8 in, 1 out]
                    n263 = local write "Error"(w378) -> ()
                    n264 = call <userlib>:"AT Get Int A.vi"("error in (no error)"=w378, "Feature"="TimestampClockFrequency", "Handle"=w375) -> ("Value"=w376:i64)  [unwired: 6 in, 2 out]
                    n265 = local write "camclockfreq"(w376) -> ()
                  }
                  frame #1 {
                    n266 = Current VI's Path() -> (path=w380:path)
                    n267 = local write "memory allocated"(TRUE ("memory allocated")) -> ()
                    n268 = call "write_parameteres_to_file1.vi"("vi path"=w380) -> ()  [unwired: 11 in]
                  }
                }
                n269 = local write "acquiring"(TRUE ("acquiring")) -> ()
              }
              frame #2 {
                n270 = local read "Handle"() -> (w383:i32)
                n271 = while {
                  shift-right: [w413] -> w384
                  shift-left: w382 -> [w414]
                  tunnel: w383 -> [w415]
                  i -> [w417]
                  stop <- w412 stop-if-true
                  n272 = stacked-sequence {
                    tunnel: w415 -> [w427 _ _]
                    tunnel: w417 -> [w420 _ w450]
                    tunnel: [_ _ w452] -> w413
                    tunnel: w414 -> [_ _ w451]
                    frame #0 {
                      w423 = u16 24578 items=["MD_FrameData"=24577, "MD_FPGATicks"=24578, "MD_FrameInfo"=24579] ("Metadata Chunk ID")
                      # "Requeue the buffer\nfor the next image"
                      # "wait for the acquisition to \nreturn and retrieve the output"
                      n273 = local read "ImageSizeBytes"() -> (w425:i64)
                      n274 = local read "ByteData"() -> (w430:u8[])
                      n275 = call <userlib>:"AT Wait Buffer A.vi"("Input buffer"=u32 0, "Timeout"=u32 10000, "Handle"=w427) -> ("error out"=w428:errorcluster, "Output buffer"=w426:u64)  [unwired: 5 in, 2 out]
                      n276 = local write "Error"(w428) -> ()
                      n277 = call <userlib>:"PointerToArrayEX.vi"("Array in"=w430, "Pointer In"=w426, "Pointer Size"=w425, "error in (no error)"=w428) -> ("Array out"=w424:u8[], "error out"=w429:errorcluster)  [unwired: 4 in]
                      n278 = local write "ByteData"(w424) -> ()
                      n279 = local read "camclockfreq"() -> (w419:i64)
                      n280 = local read "Save path"() -> (w421:path)
                      n281 = call <userlib>:"AT GetMetadata.vi"("Metadata Chunk ID"=w423, "Input buffer"=w424, "BufferSize"=w425) -> ("MetaData"=w422:i64)  [unwired: 1 in, 2 out]
                      n282 = call "write_timestamp_to_file.vi"("clock freq"=w419, "index"=w420, "metadata"=w422, "free run save path"=w421) -> ()  [unwired: 8 in]
                      n283 = call <userlib>:"AT Queue Buffer A.vi"("error in (no error)"=w429, "PtrSize"=w425, "Ptr"=w426, "Handle"=w427) -> ("error out"=w432:errorcluster)  [unwired: 6 in, 1 out]
                      n284 = local write "Error"(w432) -> ()
                    }
                    frame #1 {
                      # "Convert the buffer containing byte \ndata into an array of pixels"
                      n285 = local read "Pixel Encoding"() -> (w440:string)
                      n286 = local read "AOI Height"() -> (w437:i64)
                      n287 = local read "AOI Width"() -> (w438:i64)
                      n288 = local read "AOIStride"() -> (w441:i64)
                      n289 = local read "ByteData"() -> (w435:u8[])
                      n290 = local read "PixelData"() -> (w439:u16[])
                      n291 = call-poly <userlib>:"GetPixelData.vi"("Input buffer"=w435, "Output buffer in"=w439, "Pixel Encoding"=w440, "Stride"=w441, "Width"=w438, "Height"=w437) -> ("Output buffer out"=w434:u16[], "error out"=w436:errorcluster)  [unwired: 11 in, 1 out]
                      n292 = local write "PixelData"(w434) -> ()
                      n293 = local write "Error"(w436) -> ()
                    }
                    frame #2 {
                      w448 = T3 7 items=["Grayscale (U8)", "Grayscale (I16)", "Grayscale (SGL)", "Complex (CSG)", "RGB (U32)", "HSL (U32)", "RGB (U64)", "Grayscale (U16)"] ("Image Type")
                      # "Draw the image"
                      n294 = local read "ExposureTime (s)"() -> (w443:dbl)
                      n295 = local read "AOI Height"() -> (w454:i64)
                      n296 = local read "AOI Width"() -> (w453:i64)
                      n297 = local read "PixelData"() -> (w455:u16[])
                      n298 = call "IMAQ Create"("Image Name"="1", "Image Type"=w448) -> ("New Image"=w447:T1)  [unwired: 3 in, 1 out]
                      n299 = Reshape Array(w455, w454, w453) -> (w446:u16[][])
                      n300 = call "IMAQ ArrayToImage"("Image Pixels (U16)"=w446, "Image"=w447) -> ("Image Out"=w445:T1)  [unwired: 8 in, 1 out]
                      n301 = Greater?(x=w443, y=0.19) -> (0:w444:bool)
                      n302 = Replace Array Subset(array=w451, new element=w446, index (dim 0)=w450) -> (w452:u16[][][])  [unwired: 2 in]
                      n303 = case shown="True" w444 {
                        tunnel: w445 -> [_ w456]
                        frame False {
                        }
                        frame True {
                          n304 = local write "camera image"(w456) -> ()
                        }
                      }
                    }
                  }
                  n305 = local read "image num"() -> (w411:u64)
                  n306 = Add(x=w417, y=1) -> (x+y=w410:i32)
                  n307 = Greater Or Equal?(x=w410, y=w411) -> (x >= y?=w412:bool)
                  n308 = Not(x=w412) -> (.not. x?=w416:bool)
                  n309 = local write "acquiring"(w416) -> ()
                  n310 = local write "acquired images"(w410) -> ()
                }
                n311 = while {
                  tunnel: w384 -> [w391]
                  i -> [w397]
                  stop <- w392 stop-if-true
                  w394 = T3 7 items=["Grayscale (U8)", "Grayscale (I16)", "Grayscale (SGL)", "Complex (CSG)", "RGB (U32)", "HSL (U32)", "RGB (U64)", "Grayscale (U16)"] ("Image Type")
                  n312 = local read "Save path"() -> (w387:path)
                  n313 = Array Subset(array=w391, index (dim 0)=w397, length (dim 0)=1 ("length")) -> (w407:u16[][][])  [unwired: 4 in]
                  n314 = Add(x=w397, y=1) -> (x+y=w395:i32)
                  n315 = local read "AOI Height"() -> (w406:i64)
                  n316 = local read "AOI Width"() -> (w405:i64)
                  n317 = local read "image num"() -> (w388:u64)
                  n318 = call "IMAQ Create"("Image Name"="2", "Image Type"=w394) -> ("New Image"=w386:T1)  [unwired: 3 in, 1 out]
                  n319 = Path To String(path=w387) -> (string=w390:string)
                  n320 = Format Value(format string="%04d", value (0)=w397) -> (output string=w402:string)  [unwired: 1 in]
                  n321 = Concatenate Strings(w390, "\\" ("string"), w402, ".tif" ("string")) -> (w399:string)
                  n322 = Reshape Array(w407, w406, w405) -> (w404:u16[][])
                  n323 = call "IMAQ ArrayToImage"("Image Pixels (U16)"=w404, "Image"=w386) -> ("error out"=w403:errorcluster, "Image Out"=w385:T1)  [unwired: 8 in]
                  n324 = local write "camera image"(w385) -> ()
                  n325 = Greater Or Equal?(x=w395, y=w388) -> (x >= y?=w392:bool)
                  n326 = Not(x=w392) -> (.not. x?=w393:bool)
                  n327 = String To Path(string=w399) -> (path=w398:path)
                  n328 = local write "saving"(w393) -> ()
                  n329 = call-poly "IMAQ Write File 2"("error in (no error)"=w403, "File Path"=w398, "Image"=w385) -> ()  [unwired: 7 in, 2 out]
                }
              }
              frame #3 {
                w457 = FALSE ("memory allocated")
                # "stop acquisition"
                n330 = local read "Handle"() -> (w459:i32)
                n331 = call <userlib>:"AT Command A.vi"("Feature"="AcquisitionStop" ("Command"), "Handle"=w459) -> ()  [unwired: 8 in, 2 out]
                n332 = local write "memory allocated"(w457) -> ()
                n333 = local write "get&save image"(w457) -> ()
              }
            }
          }
          event "get&save image disk": Value Change {
            n334 = event-data() -> ()  [unwired: 1 in, 6 out]
            n335 = stacked-sequence {
              frame #0 {
                # "Get the AOI Width and Height"
                # "Get Sensor Parameters."
                n336 = local read "Handle"() -> (w463:i32)
                n337 = call <userlib>:"AT Get Int A.vi"("Feature"="AOIHeight" ("Integer feature 2"), "Handle"=w463) -> ("error out"=w462:errorcluster, "Value"=w460:i64)  [unwired: 7 in, 1 out]
                n338 = local write "AOI Height"(w460) -> ()
                n339 = local write "Error"(w462) -> ()
                n340 = call <userlib>:"AT Get Int A.vi"("error in (no error)"=w462, "Feature"="AOIWidth" ("Integer feature"), "Handle"=w463) -> ("error out"=w466:errorcluster, "Value"=w461:i64)  [unwired: 6 in, 1 out]
                n341 = local write "AOI Width"(w461) -> ()
                n342 = local write "Error"(w466) -> ()
              }
              frame #1 {
                # "Set the AOI width and height"
                # "Set the Exposure Time and Pre Amp Gain for the camera"
                # "Set Parameters."
                n343 = local read "ExposureTime (s)"() -> (w480:dbl)
                n344 = local read "Handle"() -> (w467:i32)
                n345 = local read "Error"() -> (w475:errorcluster)
                n346 = call <userlib>:"AT Set Float A.vi"("error in (no error)"=w475, "Value"=w480, "Feature"="ExposureTime" ("ExposureTime"), "Hndl"=w467) -> ("error out"=w478:errorcluster)  [unwired: 6 in, 1 out]
                n347 = local read "PreAmp Gain Control"() -> (w479:string)
                n348 = local write "Error"(w478) -> ()
                n349 = call <userlib>:"AT Set Enum String A.vi"("error in (no error)"=w478, "String"=w479, "Feature"="SimplePreAmpGainControl" ("SimplePreAmpGainControl"), "Handle"=w467) -> ("error out"=w474:errorcluster)  [unwired: 6 in, 1 out]
                n350 = local write "Error"(w474) -> ()
                n351 = local read "AOI Height"() -> (w471:i64)
                n352 = call <userlib>:"AT Set Int A.vi"("error in (no error)"=w474, "Value"=w471, "Feature"="AOIHeight" ("Integer feature"), "Handle"=w467) -> ("error out"=w472:errorcluster)  [unwired: 6 in, 1 out]
                n353 = local write "Error"(w472) -> ()
                n354 = local read "AOI Width"() -> (w470:i64)
                n355 = call <userlib>:"AT Set Int A.vi"("error in (no error)"=w472, "Value"=w470, "Feature"="AOIWidth" ("Integer feature 2"), "Handle"=w467) -> ("error out"=w473:errorcluster)  [unwired: 6 in, 1 out]
                n356 = local write "Error"(w473) -> ()
              }
              frame #2 {
                # "Centre AOI."
                n357 = local read "Centre AOI"() -> (w481:bool)
                n358 = case shown="True" w481 {
                  frame False {
                  }
                  frame True {
                    n359 = local read "AOI Height"() -> (w483:i64)
                    n360 = local read "AOI Width"() -> (w484:i64)
                    n361 = local read "Handle"() -> (w482:i32)
                    n362 = local read "Error"() -> (w485:errorcluster)
                    n363 = call <userlib>:"AT Centre AOI.vi"("error in (no error)"=w485, "AOI Width"=w484, "AOI Height"=w483, "Handle"=w482) -> ("error out"=w486:errorcluster)  [unwired: 7 in]
                    n364 = local write "Error"(w486) -> ()
                  }
                }
              }
              frame #3 {
                # "Set overlap mode,\nfaster frame rates when on"
                # "Set the pixel readout rate"
                # "Set the shutter mode,\nRolling = for fastest frame rate\nGlobal = for fast moving objects"
                # "Set the number of images that \nwill be acquired"
                # "Set the Trigger mode to 'Internal this means \nthis camera will run as fast as possible"
                # "Set the cycle mode to 'Fixed'. This tells the \ncamera to acquire a fixed number of images."
                # "Set Acquisition Mode."
                n365 = local read "Handle"() -> (w493:i32)
                n366 = local read "Error"() -> (w503:errorcluster)
                n367 = call <userlib>:"AT Set Enum String A.vi"("error in (no error)"=w503, "String"="Fixed", "Feature"="CycleMode" ("Enum feature"), "Handle"=w493) -> ("error out"=w502:errorcluster)  [unwired: 6 in, 1 out]
                n368 = local write "Error"(w502) -> ()
                n369 = local read "Trigger mode"() -> (w487:string)
                n370 = call <userlib>:"AT Set Enum String A.vi"("error in (no error)"=w502, "String"=w487, "Feature"="TriggerMode" ("Enum feature"), "Handle"=w493) -> ("error out"=w500:errorcluster)  [unwired: 6 in, 1 out]
                n371 = local write "Error"(w500) -> ()
                n372 = local read "image num"() -> (w498:u64)
                n373 = call <userlib>:"AT Set Int A.vi"("error in (no error)"=w500, "Value"=w498, "Feature"="FrameCount" ("Integer feature 2"), "Handle"=w493) -> ("error out"=w497:errorcluster)  [unwired: 6 in, 1 out]
                n374 = local read "ElectronicShutteringMode"() -> (w490:string)
                n375 = local write "Error"(w497) -> ()
                n376 = call <userlib>:"AT Set Enum String A.vi"("error in (no error)"=w497, "String"=w490, "Feature"="ElectronicShutteringMode" ("ElectronicShutteringMode"), "Handle"=w493) -> ("error out"=w496:errorcluster)  [unwired: 6 in, 1 out]
                n377 = local read "Pixel Readout Rate"() -> (w489:string)
                n378 = call <userlib>:"AT Set Enum String A.vi"("error in (no error)"=w496, "String"=w489, "Feature"="PixelReadoutRate" ("PixelReadoutRate"), "Handle"=w493) -> ("error out"=w495:errorcluster)  [unwired: 6 in, 1 out]
                n379 = local read "Overlap"() -> (w488:bool)
                n380 = call <userlib>:"AT Set Bool A.vi"("error in (no error)"=w495, "Value"=w488, "Feature"="Overlap" ("Overlap"), "Handle"=w493) -> ()  [unwired: 6 in, 2 out]
              }
              frame #4 {
                # "Set Parameters."
                n381 = local read "ExposureTime (s)"() -> (w510:dbl)
                n382 = local read "Handle"() -> (w506:i32)
                n383 = local read "Error"() -> (w507:errorcluster)
                n384 = call <userlib>:"AT Set Float A.vi"("error in (no error)"=w507, "Value"=w510, "Feature"="ExposureTime" ("ExposureTime"), "Hndl"=w506) -> ("error out"=w509:errorcluster)  [unwired: 6 in, 1 out]
                n385 = local write "Error"(w509) -> ()
              }
              frame #5 {
                n386 = local read "Trigger mode"() -> (w511:string)
                n387 = case shown="\"External\", Default" w511 {
                  frame "External", Default {
                    n388 = local read "Handle"() -> (w514:i32)
                    n389 = call <userlib>:"AT Get Float A.vi"("Feature"="FrameRate" ("FrameRate"), "Handle"=w514) -> ("Value"=w512:dbl)  [unwired: 7 in, 2 out]
                    n390 = property on="FrameRate" class="DigNum (strict)"("Value"=w512) -> ()  [unwired: 2 in, 2 out]
                  }
                  frame "Software" {
                    w517 = "FrameRate" ("FrameRate")
                    n391 = local read "Handle"() -> (w516:i32)
                    n392 = call <userlib>:"AT Get Float Max A.vi"("Feature"=w517, "Handle"=w516) -> ("error out"=w520:errorcluster, "MaxValue"=w519:dbl)  [unwired: 7 in, 1 out]
                    n393 = call <userlib>:"AT Set Float A.vi"("error in (no error)"=w520, "Value"=w519, "Feature"=w517, "Hndl"=w516) -> ("error out"=w518:errorcluster)  [unwired: 6 in, 1 out]
                    n394 = call <userlib>:"AT Get Float A.vi"("error in (no error)"=w518, "Feature"=w517, "Handle"=w516) -> ("Value"=w515:dbl)  [unwired: 6 in, 2 out]
                    n395 = property on="FrameRate" class="DigNum (strict)"("Value"=w515) -> ()  [unwired: 2 in, 2 out]
                  }
                  frame "Internal" {
                    w523 = "FrameRate" ("FrameRate")
                    n396 = local read "Handle"() -> (w522:i32)
                    n397 = call <userlib>:"AT Get Float Max A.vi"("Feature"=w523, "Handle"=w522) -> ("error out"=w526:errorcluster, "MaxValue"=w525:dbl)  [unwired: 7 in, 1 out]
                    n398 = call <userlib>:"AT Set Float A.vi"("error in (no error)"=w526, "Value"=w525, "Feature"=w523, "Hndl"=w522) -> ("error out"=w524:errorcluster)  [unwired: 6 in, 1 out]
                    n399 = call <userlib>:"AT Get Float A.vi"("error in (no error)"=w524, "Feature"=w523, "Handle"=w522) -> ("Value"=w521:dbl)  [unwired: 6 in, 2 out]
                    n400 = property on="FrameRate" class="DigNum (strict)"("Value"=w521) -> ()  [unwired: 2 in, 2 out]
                  }
                }
              }
              frame #6 {
                # "Get settings and Create Buffers."
                n401 = stacked-sequence {
                  frame #0 {
                    w535 = "PixelEncoding" ("Enum feature")
                    # "Get the frame rate the camera will run at"
                    # "Retrieve a string containing \nthe current pixel encoding"
                    # "Stride of the\nimage in pixels"
                    # "Size of the\nimages in Bytes.\nHeight*Stride*BytesPerPixel"
                    n402 = local read "Error"() -> (w532:errorcluster)
                    n403 = local read "Handle"() -> (w529:i32)
                    n404 = call <userlib>:"AT Get Int A.vi"("error in (no error)"=w532, "Feature"="AOIStride" ("Integer feature"), "Handle"=w529) -> ("error out"=w538:errorcluster, "Value"=w542:i64)  [unwired: 6 in, 1 out]
                    n405 = call <userlib>:"AT Get Int A.vi"("error in (no error)"=w538, "Feature"="ImageSizeBytes" ("Integer feature"), "Handle"=w529) -> ("error out"=w537:errorcluster, "Value"=w541:i64)  [unwired: 6 in, 1 out]
                    n406 = call <userlib>:"AT Get Enum Index A.vi"("error in (no error)"=w537, "Feature"=w535, "Handle"=w529) -> ("error out"=w536:errorcluster, "Value"=w534:i32)  [unwired: 6 in, 1 out]
                    n407 = call <userlib>:"AT Get Enum String By Index A.vi"("error in (no error)"=w536, "Index"=w534, "Feature"=w535, "Handle"=w529) -> ("error out"=w528:errorcluster, "String"=w533:string)  [unwired: 5 in, 1 out]
                    n408 = call <userlib>:"AT Get Float A.vi"("error in (no error)"=w528, "Feature"="FrameRate", "Handle"=w529) -> ("error out"=w530:errorcluster, "Value"=w527:dbl)  [unwired: 6 in, 1 out]
                    n409 = local write "ImageSizeBytes"(w541) -> ()
                    n410 = local write "Pixel Encoding"(w533) -> ()
                    n411 = local write "AOIStride"(w542) -> ()
                    n412 = local write "Error"(w538) -> ()
                    n413 = local write "Error"(w537) -> ()
                    n414 = local write "Error"(w536) -> ()
                    n415 = local write "Error"(w528) -> ()
                    n416 = local write "FrameRate"(w527) -> ()
                    n417 = local write "Error"(w530) -> ()
                  }
                  frame #1 {
                    w544 = u8 0
                    # "Test for timestamp"
                    # "Buffer to hold the raw data that comes off the camera"
                    n418 = local read "ImageSizeBytes"() -> (w543:i64)
                    n419 = Initialize Array(w544, w543) -> (w545:u8[])
                    n420 = Initialize Array(w544, w543) -> (w546:u8[])
                    n421 = local write "ByteData"(w545) -> ()
                    n422 = local write "PixelData"(w546) -> ()
                  }
                  frame #2 {
                    # "Create 300MB of buffers - this allows sufficient memory to retrieve \ndata into while files are written to disk"
                    # "Clear any buffers \non the camera"
                    n423 = local read "ImageSizeBytes"() -> (w550:i64)
                    n424 = local read "Error"() -> (w557:errorcluster)
                    n425 = local read "Handle"() -> (w555:i32)
                    n426 = Multiply(x=300, y=1024) -> (x*y=w553:i32)
                    n427 = Multiply(x=w553, y=1024) -> (x*y=w549:i32)
                    n428 = call <userlib>:"AT Clear All Buffers A.vi"("error in (no error)"=w557, "Handle"=w555) -> ("error out"=w556:errorcluster)  [unwired: 8 in, 1 out]
                    n429 = local write "Error"(w556) -> ()
                    n430 = Divide(x=w549, y=w550) -> (x/y=w548:dbl)
                    n431 = To Long Integer(number=w548) -> (32bit integer=w547:i32)
                    n432 = for {
                      N: w547 -> [_]
                      tunnel: w556 -> [w560]
                      tunnel: w555 -> [w559]
                      i -> [w558]
                      # "Create a buffer to store 1 image coming off the camera"
                      n433 = local read "ImageSizeBytes"() -> (w562:i64)
                      n434 = call <userlib>:"AT Create Buffer A.vi"("error in (no error)"=w560, "Buffer"=w558, "Size"=w562, "Handle"=w559) -> ("error out"=w563:errorcluster, "Buffer out"=w564:u64)  [unwired: 5 in, 1 out]
                      n435 = local write "Error"(w563) -> ()
                      n436 = call <userlib>:"AT Queue Buffer A.vi"("error in (no error)"=w563, "PtrSize"=w562, "Ptr"=w564, "Handle"=w559) -> ("error out"=w561:errorcluster)  [unwired: 6 in, 1 out]
                      n437 = local write "Error"(w561) -> ()
                    }
                  }
                }
              }
              frame #7 {
                # "2. Queue images as they arrive off the camera"
                # "Acquire"
                n438 = flat-sequence {
                  frame #0 {
                    w570 = "AcquisitionStart"  # Command
                    # "Start the acquisition"
                    n439 = local read "Handle"() -> (w568:i32)
                    n440 = local read "Error"() -> (w571:errorcluster)
                    n441 = call <userlib>:"AT Command A.vi"("error in (no error)"=w571, "Feature"=w570, "Handle"=w568) -> ("error out"=w566:errorcluster)  [unwired: 7 in, 1 out]
                    n442 = Current VI's Path() -> (path=w567:path)
                    n443 = local write "Error"(w566) -> ()
                    n444 = call "write_parameteres_to_file1.vi"("error"=w566, "vi path"=w567) -> ()  [unwired: 10 in]
                    n445 = call <userlib>:"AT Get Int A.vi"("error in (no error)"=w566, "Feature"="TimestampClockFrequency", "Handle"=w568) -> ("Value"=w565:i64)  [unwired: 6 in, 2 out]
                    n446 = local write "camclockfreq"(w565) -> ()
                  }
                  frame #1 {
                    n447 = local write "memory allocated"(TRUE ("memory allocated")) -> ()
                    n448 = local write "acquiring"(TRUE ("acquiring")) -> ()
                  }
                }
              }
              frame #8 {
                n449 = local read "image num"() -> (w574:u64)
                n450 = local read "image num"() -> (w581:u64)
                n451 = local read "Trigger mode"() -> (w580:string)
                n452 = local read "Handle"() -> (w575:i32)
                n453 = Obtain Queue(max queue size (-1, unlimited)=w574, name (unnamed)="Data", element data type=u64 0) -> (queue out=w584:refnum<queue>, error out=w585:errorcluster)  [unwired: 2 in, 1 out]
                n454 = Obtain Queue(max queue size (-1, unlimited)=w581, name (unnamed)="Data", element data type=u64 0) -> (queue out=w583:refnum<queue>)  [unwired: 2 in, 2 out]
                n455 = while {
                  tunnel: w585 -> [w655]
                  tunnel: w584 -> [w654]
                  tunnel: [w651] -> w582
                  i -> [w621]
                  stop <- w644 stop-if-true
                  w637 = T3 7 items=["Grayscale (U8)", "Grayscale (I16)", "Grayscale (SGL)", "Complex (CSG)", "RGB (U32)", "HSL (U32)", "RGB (U64)", "Grayscale (U16)"] ("Image Type")
                  # "3. Write out a file for each image coming off the camera"
                  n456 = local read "ImageSizeBytes"() -> (w645:i64)
                  n457 = Dequeue Element(queue=w654, timeout in ms (-1)=10000, error in (no error)=w655) -> (queue out=w651:refnum<queue>, element=w646:u64, error out=w647:errorcluster)  [unwired: 1 out]
                  n458 = local read "ByteData"() -> (w648:u8[])
                  n459 = local read "Pixel Encoding"() -> (w640:string)
                  n460 = local read "AOI Height"() -> (w633:i64)
                  n461 = local read "AOI Width"() -> (w632:i64)
                  n462 = local read "AOIStride"() -> (w639:i64)
                  n463 = local read "PixelData"() -> (w641:u16[])
                  n464 = call <userlib>:"PointerToArrayEX.vi"("Array in"=w648, "Pointer In"=w646, "Pointer Size"=w645, "error in (no error)"=w647) -> ("Array out"=w642:u8[], "error out"=w620:errorcluster)  [unwired: 4 in]
                  n465 = local read "Save path"() -> (w626:path)
                  n466 = call-poly <userlib>:"GetPixelData.vi"("Input buffer"=w642, "Output buffer in"=w641, "Pixel Encoding"=w640, "Stride"=w639, "error in (no error)"=w620, "Width"=w632, "Height"=w633) -> ("Output buffer out"=w634:u16[], "error out"=w619:errorcluster)  [unwired: 10 in, 1 out]
                  n467 = local read "image num"() -> (w649:u64)
                  n468 = call "IMAQ Create"("Image Name"="s", "Image Type"=w637) -> ("New Image"=w635:T1, "error out"=w636:errorcluster)  [unwired: 3 in]
                  n469 = Reshape Array(w634, w633, w632) -> (w631:u16[][])
                  n470 = Increment(x=w621) -> (x+1=w650:i32)
                  n471 = local read "Handle"() -> (w652:i32)
                  n472 = Path To String(path=w626) -> (string=w630:string)
                  n473 = call "IMAQ ArrayToImage"("Image Pixels (U16)"=w631, "error in (no error)"=w636, "Image"=w635) -> ("Image Out"=w623:T1)  [unwired: 7 in, 1 out]
                  n474 = Format Value(format string="%04d", value (0)=w621) -> (output string=w629:string)  [unwired: 1 in]
                  n475 = Concatenate Strings(w630, "\\" ("string"), w629, ".tif" ("string")) -> (w625:string)
                  n476 = Equal?(x=w650, y=w649) -> (x = y?=w644:bool)
                  n477 = Not(x=w644) -> (.not. x?=w643:bool)
                  n478 = local write "saving"(w643) -> ()
                  n479 = String To Path(string=w625) -> (path=w624:path)
                  n480 = call-poly "IMAQ Write File 2"("File Path"=w624, "Image"=w623) -> ()  [unwired: 8 in, 2 out]
                  n481 = call <userlib>:"AT Queue Buffer A.vi"("error in (no error)"=w619, "PtrSize"=w645, "Ptr"=w646, "Handle"=w652) -> ()  [unwired: 6 in, 2 out]
                }
                n482 = while {
                  tunnel: w575 -> [w599]
                  tunnel: w583 -> [w606]
                  tunnel: w581 -> [w605]
                  tunnel: w580 -> [w601]
                  i -> [w589]
                  stop <- w598 stop-if-true
                  w591 = u16 24578 items=["MD_FrameData"=24577, "MD_FPGATicks"=24578, "MD_FrameInfo"=24579] ("Metadata Chunk ID")
                  n483 = case shown="\"Software\"" w601 {
                    tunnel: [w613 w616 w618] -> w600
                    tunnel: w599 -> [_ w615 _]
                    frame "Internal", Default {
                      n484 = local read "Error"() -> (w613:errorcluster)
                    }
                    frame "Software" {
                      n485 = local read "Error"() -> (w614:errorcluster)
                      n486 = call <userlib>:"AT Command A.vi"("error in (no error)"=w614, "Feature"="SoftwareTrigger" ("Command"), "Handle"=w615) -> ("error out"=w616:errorcluster)  [unwired: 7 in, 1 out]
                    }
                    frame "External" {
                      n487 = local read "Error"() -> (w618:errorcluster)
                    }
                  }
                  n488 = local read "ImageSizeBytes"() -> (w594:i64)
                  n489 = call <userlib>:"AT Wait Buffer A.vi"("error in (no error)"=w600, "Input buffer"=u64 0, "Timeout"=u32 2000, "Handle"=w599) -> ("error out"=w596:errorcluster, "Output buffer"=w602:u64)  [unwired: 4 in, 2 out]
                  n490 = local read "camclockfreq"() -> (w588:i64)
                  n491 = local read "PixelData"() -> (w603:u16[])
                  n492 = local read "Save path"() -> (w587:path)
                  n493 = call <userlib>:"PointerToArrayEX.vi"("Array in"=w603, "Pointer In"=w602, "Pointer Size"=w594, "error in (no error)"=w596) -> ("Array out"=w593:u8[], "error out"=w592:errorcluster)  [unwired: 4 in]
                  n494 = local write "Error"(w596) -> ()
                  n495 = call <userlib>:"AT GetMetadata.vi"("Metadata Chunk ID"=w591, "error in (no error)"=w592, "Input buffer"=w593, "BufferSize"=w594) -> ("MetaData"=w590:i64, "error out"=w586:errorcluster)  [unwired: 1 out]
                  n496 = call "write_timestamp_to_file.vi"("clock freq"=w588, "index"=w589, "metadata"=w590, "free run save path"=w587) -> ()  [unwired: 8 in]
                  n497 = case shown="No Error" w586 {
                    tunnel: w606 -> [w611 _]
                    tunnel: [w610 w612] -> w604
                    tunnel: w602 -> [w609 _]
                    tunnel: w589 -> [w608 _]
                    frame No Error {
                      n498 = Enqueue Element(queue=w611, element=w609) -> ()  [unwired: 2 in, 3 out]
                      n499 = Increment(x=w608) -> (x+1=w610:i32)
                      n500 = local write "acquired images"(w610) -> ()
                    }
                    frame Error {
                      n501 = local read "image num"() -> (w612:u64)
                    }
                  }
                  n502 = Equal?(x=w605, y=w604) -> (x = y?=w598:bool)
                  n503 = Not(x=w598) -> (.not. x?=w597:bool)
                  n504 = local write "acquiring"(w597) -> ()
                }
                n505 = Release Queue(queue=w582) -> ()  [unwired: 2 in, 3 out]
              }
              frame #9 {
                n506 = flat-sequence {
                  frame #0 {
                    # "Stop an acquisition if still running"
                    n507 = local read "Handle"() -> (w657:i32)
                    n508 = call <userlib>:"AT Command A.vi"("Feature"="AcquisitionStop" ("Command"), "Handle"=w657) -> ()  [unwired: 8 in, 2 out]
                  }
                  frame #1 {
                    w658 = FALSE ("get&save image disk")
                    # "Clear any buffers \non the camera"
                    n509 = local read "Error"() -> (w659:errorcluster)
                    n510 = local read "Handle"() -> (w661:i32)
                    n511 = call <userlib>:"AT Clear All Buffers A.vi"("error in (no error)"=w659, "Handle"=w661) -> ("error out"=w660:errorcluster)  [unwired: 8 in, 1 out]
                    n512 = local write "memory allocated"(w658) -> ()
                    n513 = local write "get&save image disk"(w658) -> ()
                    n514 = local write "Error"(w660) -> ()
                  }
                }
              }
            }
          }
        }
        n515 = local read "Stop"() -> (w281:bool)
      }
      n516 = while {
        stop <- w46 stop-if-true
        n517 = local read "show temperature"() -> (w45:bool)
        n518 = case shown="True" w45 {
          frame False {
          }
          frame True {
            n519 = local read "Handle"() -> (w49:i32)
            n520 = call <userlib>:"AT Get Float A.vi"("Feature"="SensorTemperature" ("SensorTemperature"), "Handle"=w49) -> ("Value"=→"camera temperature(℃)":dbl)  [unwired: 7 in, 2 out]
          }
        }
        n521 = local read "Stop"() -> (w46:bool)
        n522 = Wait (ms)(milliseconds to wait=u32 100) -> ()  [unwired: 1 out]
      }
      n523 = while {
        stop <- w175 stop-if-true
        # "matlab related events"
        n524 = event shown="[2] \"call matlab for acq\": Value Change" {
          selector: _ -> [_ _ _]
          dyn-events: _ -> [_ _ _]
          timeout: 1 -> [_ _ _]
          event Timeout {
            n525 = event-data() -> ()  [unwired: 1 in, 3 out]
          }
          event "call matlab for cali": Value Change {
            n526 = event-data() -> ()  [unwired: 1 in, 6 out]
            n527 = stacked-sequence {
              frame #0 {
                n528 = local read "illumination delay deg"() -> (w182:dbl)
                n529 = local read "illumination last deg"() -> (w181:dbl)
                n530 = local read "dmd pattern num"() -> (w183:u64)
                n531 = local read "dmd pattern num"() -> (w177:u64)
                n532 = local read "cali pattern path"() -> (w188:path)
                n533 = local read "load cali pattern"() -> (w187:bool)
                n534 = local read "signal time (ms)"() -> (w184:dbl)
                n535 = local read "Frame number"() -> (w178:i32)
                n536 = local read "dmd delay deg"() -> (w185:dbl)
                n537 = local read "cam delay deg"() -> (w186:dbl)
                n538 = Multiply(x=w178, y=w177) -> (x*y=w176:u64)
                n539 = local write "load patterns"(w187) -> ()
                n540 = local write "pattern path"(w188) -> ()
                n541 = call "matlab_for_calibration.vi"("illumination last degree"=w181, "illumination delay degree"=w182, "dmd pattern num"=w183, "camera delay degree"=w186, "dmd delay degree"=w185, "signal_time(ms)"=w184) -> ("exposure time(s)"=w190:dbl, "sample num"=w191:dbl, "DO signal"=w189:dbl[][], "sample rate"=w180:dbl, "dmd_picture_time(us)"=w179:dbl)  [unwired: 1 in]
                n542 = local write "image num"(w176) -> ()
                n543 = local write "ExposureTime (s)"(w190) -> ()
                n544 = local write "DO signal"(w189) -> ()
                n545 = local write "DO sample num"(w191) -> ()
                n546 = local write "dmd_picture_time"(w179) -> ()
                n547 = local write "sample rate"(w180) -> ()
              }
              frame #1 {
                n548 = local write "call matlab for cali"(FALSE ("call matlab for cali")) -> ()
              }
            }
          }
          event "call matlab for acq": Value Change {
            n549 = event-data() -> ()  [unwired: 1 in, 6 out]
            n550 = stacked-sequence {
              frame #0 {
                n551 = local read "illumination delay deg"() -> (w196:dbl)
                n552 = local read "illumination last deg"() -> (w195:dbl)
                n553 = local read "acq pattern path"() -> (w205:path)
                n554 = local read "acq signal time (ms)"() -> (w198:dbl)
                n555 = local read "dmd pattern num"() -> (w197:u64)
                n556 = local read "Frame number"() -> (w206:i32)
                n557 = local read "dmd delay deg"() -> (w199:dbl)
                n558 = local read "cam delay deg"() -> (w200:dbl)
                n559 = local write "image num"(w206) -> ()
                n560 = local write "load patterns"(TRUE) -> ()
                n561 = local write "pattern path"(w205) -> ()
                n562 = call "matlab_for_acquisition.vi"("illumination last degree"=w195, "illumination delay degree"=w196, "dmd pattern num"=w197, "camera delay degree"=w200, "dmd delay degree"=w199, "signal_time(ms)"=w198) -> ("exposure time"=w201:dbl, "sample num"=w203:dbl, "DO signal"=w202:dbl[][], "sample rate"=w204:dbl, "dmd_picture_time"=w193:dbl)  [unwired: 1 in]
                n563 = local write "DO sample num"(w203) -> ()
                n564 = local write "ExposureTime (s)"(w201) -> ()
                n565 = local write "dmd_picture_time"(w193) -> ()
                n566 = local write "sample rate"(w204) -> ()
                n567 = local write "DO signal"(w202) -> ()
              }
              frame #1 {
                n568 = local write "call matlab for acq"(FALSE ("call matlab for acq")) -> ()
              }
            }
          }
        }
        n569 = local read "Stop"() -> (w175:bool)
      }
      n570 = while {
        stop <- w111 stop-if-true
        n571 = event shown="[0] \"start cali\": Value Change" {
          selector: _ -> [_ _ _ _ _ _]
          dyn-events: _ -> [_ _ _ _ _ _]
          timeout: 1 -> [_ _ _ _ _ _]
          event "start cali": Value Change {
            # "start cali"
            n572 = event-data() -> ()  [unwired: 1 in, 6 out]
            n573 = local read "rotary voltage"() -> (w114:dbl)
            n574 = Greater?(x=w114, y=0.0) -> (0:w112:bool)
            n575 = case shown="True" w112 {
              frame False {
              }
              frame True {
                n576 = stacked-sequence {
                  frame #0 {
                    n577 = local write "Start.Retriggerable"(TRUE ("Start.Retriggerable")) -> ()
                    n578 = property on="call matlab for cali" class="Bool (strict)"("Val(Sgnl)"=TRUE ("Value (Signaling)")) -> ()  [unwired: 2 in, 2 out]
                    n579 = property on="dmd projection" class="Bool (strict)"("Val(Sgnl)"=TRUE ("Value (Signaling)")) -> ()  [unwired: 2 in, 2 out]
                  }
                  frame #1 {
                    n580 = while {
                      stop <- w118 continue-if-true
                      n581 = local read "call matlab for cali"() -> (w118:bool)
                    }
                  }
                  frame #2 {
                    n582 = property on="get&save image" class="Bool (strict)"("Val(Sgnl)"=TRUE ("Value (Signaling)")) -> ()  [unwired: 2 in, 2 out]
                  }
                  frame #3 {
                    n583 = while {
                      stop <- w120 stop-if-true
                      n584 = local read "memory allocated"() -> (w120:bool)
                    }
                  }
                  frame #4 {
                    n585 = property on="waveform generation" class="Bool (strict)"("Val(Sgnl)"=TRUE ("Value (Signaling)")) -> ()  [unwired: 2 in, 2 out]
                  }
                  frame #5 {
                    n586 = while {
                      stop <- w122 continue-if-true
                      n587 = local read "acquiring"() -> (w122:bool)
                    }
                  }
                  frame #6 {
                    n588 = property on="dmd projection" class="Bool (strict)"("Val(Sgnl)"=FALSE ("Value (Signaling)")) -> ()  [unwired: 2 in, 2 out]
                    n589 = property on="waveform generation" class="Bool (strict)"("Val(Sgnl)"=FALSE ("Value (Signaling)")) -> ()  [unwired: 2 in, 2 out]
                    n590 = Wait (ms)(milliseconds to wait=u32 100) -> ()  [unwired: 1 out]
                  }
                  frame #7 {
                    n591 = call "led_on_off.vi"("data"=FALSE) -> ()  [unwired: 11 in]
                  }
                  frame #8 {
                    n592 = while {
                      stop <- w127 continue-if-true
                      n593 = local read "memory allocated"() -> (w127:bool)
                    }
                  }
                }
              }
            }
          }
          event "waveform only": Value Change {
            # "start cali"
            n594 = event-data() -> ("NewVal"=w128:bool)  [unwired: 1 in, 5 out]
            n595 = case shown="True" w128 {
              frame False {
                n596 = property on="dmd projection" class="Bool (strict)"("Val(Sgnl)"=FALSE ("Value (Signaling)")) -> ()  [unwired: 2 in, 2 out]
                n597 = property on="waveform generation" class="Bool (strict)"("Val(Sgnl)"=FALSE ("Value (Signaling)")) -> ()  [unwired: 2 in, 2 out]
              }
              frame True {
                n598 = stacked-sequence {
                  frame #0 {
                    n599 = local write "Start.Retriggerable"(TRUE ("Start.Retriggerable")) -> ()
                    n600 = property on="call matlab for cali" class="Bool (strict)"("Val(Sgnl)"=TRUE ("Value (Signaling)")) -> ()  [unwired: 2 in, 2 out]
                    n601 = property on="dmd projection" class="Bool (strict)"("Val(Sgnl)"=TRUE ("Value (Signaling)")) -> ()  [unwired: 2 in, 2 out]
                  }
                  frame #1 {
                    n602 = while {
                      stop <- w134 stop-if-true
                      n603 = local read "call matlab for cali"() -> (w135:bool)
                      n604 = Not(x=w135) -> (.not. x?=w134:bool)
                    }
                  }
                  frame #2 {
                    n605 = property on="waveform generation" class="Bool (strict)"("Val(Sgnl)"=TRUE ("Value (Signaling)")) -> ()  [unwired: 2 in, 2 out]
                  }
                }
              }
            }
          }
          event "acq waveform only": Value Change {
            n606 = event-data() -> ("NewVal"=w137:bool)  [unwired: 1 in, 5 out]
            n607 = case shown="True" w137 {
              frame False {
                n608 = property on="dmd projection" class="Bool (strict)"("Val(Sgnl)"=FALSE ("Value (Signaling)")) -> ()  [unwired: 2 in, 2 out]
                n609 = property on="waveform generation" class="Bool (strict)"("Val(Sgnl)"=FALSE ("Value (Signaling)")) -> ()  [unwired: 2 in, 2 out]
              }
              frame True {
                n610 = stacked-sequence {
                  frame #0 {
                    n611 = property on="dmd projection" class="Bool (strict)"("Val(Sgnl)"=TRUE ("Value (Signaling)")) -> ()  [unwired: 2 in, 2 out]
                    n612 = property on="call matlab for acq" class="Bool (strict)"("Val(Sgnl)"=TRUE ("Value (Signaling)")) -> ()  [unwired: 2 in, 2 out]
                    n613 = local write "Start.Retriggerable"(TRUE ("Start.Retriggerable")) -> ()
                  }
                  frame #1 {
                    n614 = while {
                      stop <- w143 stop-if-true
                      n615 = local read "call matlab for acq"() -> (w144:bool)
                      n616 = Not(x=w144) -> (.not. x?=w143:bool)
                    }
                  }
                  frame #2 {
                    n617 = property on="waveform generation" class="Bool (strict)"("Val(Sgnl)"=TRUE ("Value (Signaling)")) -> ()  [unwired: 2 in, 2 out]
                  }
                }
              }
            }
          }
          event "start acq": Value Change {
            # "start cali"
            n618 = event-data() -> ()  [unwired: 1 in, 6 out]
            n619 = local read "rotary voltage"() -> (w148:dbl)
            n620 = Greater?(x=w148, y=0.0) -> (0:w146:bool)
            n621 = case shown="True" w146 {
              frame False {
              }
              frame True {
                n622 = stacked-sequence {
                  frame #0 {
                    n623 = local write "Start.Retriggerable"(TRUE ("Start.Retriggerable")) -> ()
                    n624 = property on="call matlab for acq" class="Bool (strict)"("Val(Sgnl)"=TRUE ("Value (Signaling)")) -> ()  [unwired: 2 in, 2 out]
                    n625 = property on="dmd projection" class="Bool (strict)"("Val(Sgnl)"=TRUE ("Value (Signaling)")) -> ()  [unwired: 2 in, 2 out]
                  }
                  frame #1 {
                    n626 = while {
                      stop <- w152 stop-if-true
                      n627 = local read "call matlab for acq"() -> (w153:bool)
                      n628 = Not(x=w153) -> (.not. x?=w152:bool)
                    }
                  }
                  frame #2 {
                    n629 = local read "save to disk"() -> (w154:bool)
                    n630 = case shown="False" w154 {
                      frame False {
                        n631 = property on="get&save image" class="Bool (strict)"("Val(Sgnl)"=TRUE ("Value (Signaling)")) -> ()  [unwired: 2 in, 2 out]
                      }
                      frame True {
                        n632 = property on="get&save image disk" class="Bool (strict)"("Val(Sgnl)"=TRUE ("Value (Signaling)")) -> ()  [unwired: 2 in, 2 out]
                      }
                    }
                  }
                  frame #3 {
                    n633 = while {
                      stop <- w157 stop-if-true
                      n634 = local read "memory allocated"() -> (w157:bool)
                    }
                  }
                  frame #4 {
                    n635 = property on="waveform generation" class="Bool (strict)"("Val(Sgnl)"=TRUE ("Value (Signaling)")) -> ()  [unwired: 2 in, 2 out]
                  }
                  frame #5 {
                    n636 = while {
                      stop <- w159 continue-if-true
                      n637 = local read "acquiring"() -> (w159:bool)
                    }
                  }
                  frame #6 {
                    n638 = property on="dmd projection" class="Bool (strict)"("Val(Sgnl)"=FALSE ("Value (Signaling)")) -> ()  [unwired: 2 in, 2 out]
                    n639 = property on="waveform generation" class="Bool (strict)"("Val(Sgnl)"=FALSE ("Value (Signaling)")) -> ()  [unwired: 2 in, 2 out]
                  }
                  frame #7 {
                    n640 = flat-sequence {
                      frame #0 {
                        n641 = local read "acq signal time (ms)"() -> (w162:dbl)
                        n642 = Wait (ms)(milliseconds to wait=w162) -> ()  [unwired: 1 out]
                      }
                      frame #1 {
                        n643 = call "led_on_off.vi"("data"=FALSE) -> ()  [unwired: 11 in]
                      }
                    }
                  }
                  frame #8 {
                    n644 = while {
                      stop <- w164 continue-if-true
                      n645 = local read "memory allocated"() -> (w164:bool)
                    }
                  }
                }
              }
            }
          }
          event "free run save": Value Change {
            # "start cali"
            n646 = event-data() -> ()  [unwired: 1 in, 6 out]
            n647 = stacked-sequence {
              frame #0 {
                n648 = local read "Frame number"() -> (w165:i32)
                n649 = local write "image num"(w165) -> ()
              }
              frame #1 {
                n650 = local read "save to disk"() -> (w166:bool)
                n651 = case shown="True" w166 {
                  frame False {
                    n652 = property on="get&save image" class="Bool (strict)"("Val(Sgnl)"=TRUE ("Value (Signaling)")) -> ()  [unwired: 2 in, 2 out]
                  }
                  frame True {
                    n653 = property on="get&save image disk" class="Bool (strict)"("Val(Sgnl)"=TRUE ("Value (Signaling)")) -> ()  [unwired: 2 in, 2 out]
                  }
                }
              }
              frame #2 {
                n654 = while {
                  stop <- w169 stop-if-true
                  n655 = local read "memory allocated"() -> (w169:bool)
                }
              }
              frame #3 {
                n656 = while {
                  stop <- w170 continue-if-true
                  n657 = local read "Handle"() -> (w172:i32)
                  n658 = local read "memory allocated"() -> (w170:bool)
                  n659 = call <userlib>:"AT Command A.vi"("Feature"="SoftwareTrigger" ("Command"), "Handle"=w172) -> ("error out"=w171:errorcluster)  [unwired: 8 in, 1 out]
                  n660 = local write "Error"(w171) -> ()
                }
              }
            }
          }
          event Timeout {
            n661 = event-data() -> ()  [unwired: 1 in, 3 out]
          }
        }
        n662 = local read "Stop"() -> (w111:bool)
      }
      n663 = while {
        stop <- w672 stop-if-true
        # "measure rotary stage speed"
        n664 = local read "starting edge"() -> (w667:i32)
        n665 = local read "Stop/Start"() -> (w670:bool)
        n666 = local read "rotary out"() -> (w671:tag)
        n667 = local read "counter"() -> (w668:tag)
        n668 = call "measure_rotary_stage_speed.vi"("Stop/Start"=w670, "starting edge"=w667, "rotary out"=w671, "counter channel"=w668) -> ("stage speed"=w666:dbl)
        n669 = Divide(x=1000.0, y=w666) -> (x/y=w665:dbl)
        n670 = local read "Stop"() -> (w672:bool)
        n671 = local write "rps"(w666) -> ()
        n672 = local write "T(ms)"(w665) -> ()
      }
      n673 = while {
        stop <- w664 stop-if-true
        # "monitor waveform"
        n674 = local read "Stop"() -> (w663:bool)
        n675 = call "DAQ Assistant"("stop (F)"=w663) -> ("data"=→"Waveform Graph":dynamicdata, "stopped"=w664:bool)  [unwired: 15 in, 2 out]
      }
    }
  }
